vi "PWM to Speed Test.vi"() -> ()   [LabVIEW 2015]
panel:
  in  "stop":bool
  in  "PWM":dbl min=0.0 max=0.12 step=0.005
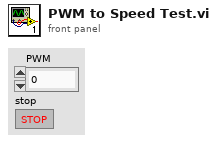
[diagram p1: front panel]
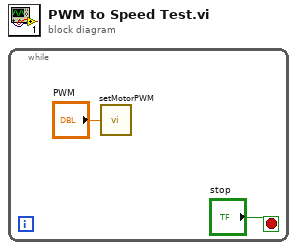
[diagram p0: block diagram]
diagram:
  n1 = while {
    stop <- "stop" stop-if-true
    n2 = call "setMotorPWM.vi"("Numeric"="PWM") -> ()
  }
